vi "RankNodes.vi"(9 "VI_AST in":refnum<class "VI_AST.lvclass">) -> (3 "VI_AST out":refnum<class "VI_AST.lvclass">)   [LabVIEW 2014, in "VI_AST.lvclass"]
uses:
  VI_AST.lvclass
  VI_AST.lvclass/VI_AST.ctl
  DAG/DAG/DAG.lvclass
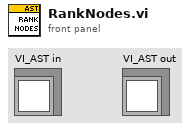
[diagram p1: front panel]
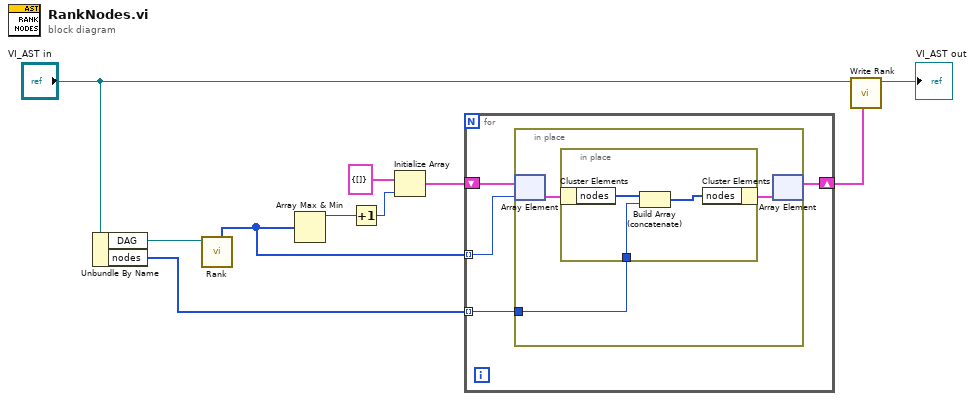
[diagram p0: block diagram]
diagram:
  n1 = Unbundle By Name("VI_AST in") -> ("DAG"=w10:refnum<class "DAG.lvclass">, "nodes"=w4:i32[])
  n2 = call "Rank.vi"("DAG in"=w10) -> ("rank"=w5:i32[])  [unwired: 8 in]
  n3 = Array Max & Min(array=w5) -> (max value=w8:i32)  [unwired: 3 out]
  n4 = Increment(x=w8) -> (x+1=w7:i32)
  n5 = Initialize Array(cluster{"nodes":i32[]} {"nodes"=[]}, w7) -> (w6:cluster{"nodes":i32[]}[])
  n6 = for {
    shift-right: [w12] -> w3
    shift-left: w6 -> [w14]
    tunnel: w4 -> [w11] mode=indexing
    tunnel: w5 -> [w13] mode=indexing
    n7 = in-place {
      in-place-border: w11 -> [w15]
      n8 = in-place-array #1(w14, w13) -> (w17:cluster{"nodes":i32[]})
      n9 = in-place {
        in-place-border: w15 -> [w18]
        n10 = in-place-cluster #2(w17) -> ("nodes"=w20:i32[])
        n11 = Build Array (concatenate)(w20, w18) -> (w19:i32[])
        n12 = in-place-cluster #2("nodes"=w19) -> (w16:cluster{"nodes":i32[]})
      }
      n13 = in-place-array #1(w16) -> (w12:cluster{"nodes":i32[]}[])  [unwired: 1 out]
    }
  }
  n14 = call "Write Rank.vi"("Rank"=w3, "VI_AST in"="VI_AST in") -> ("VI_AST out"=→"VI_AST out":refnum<class "VI_AST.lvclass">)  [unwired: 7 in]
